vi "dsdll_output_set_volume.vi"(8 "error in":errorcluster, 9 "panning (0: balanced)":i32 min=-10000 max=10000 step=1, 10 "volume (0: full)":i32 min=-10000 max=0 step=1, 11 "dsdll instance in":T1={"dsdll path"=path "E:/LVprog/DirectSoundDLL/dsdll.dll", "dsdll handle"=[], "output devices"=[], "capture devices"=[]}) -> (0 "error out":errorcluster, 3 "dsdll instance out":T1)   [LabVIEW 2020, in "dsdll.lvlib"]
doc: "Call to set volume and panning of the playback. 'volume' range is {-10000 to 0}, where -10000 is equal to -100dB and 0 is 0dB (max volume). 'panning' range is {-10000 to +10000} where 10000 is equal to 100dB."
uses:
  dsdll.lvlib
  dsdll_instance.ctl
  dsdll_device_record.ctl
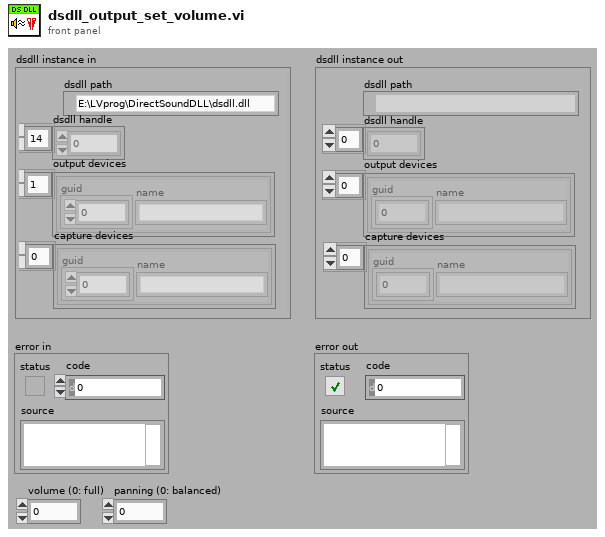
[diagram p1: front panel]
types:
  T1 = typedef "dsdll.lvlib/dsdll_instance.ctl" = cluster{"dsdll path":path, "dsdll handle":u8[], "output devices":T2[], "capture devices":T2[]}
  T2 = typedef "dsdll.lvlib/dsdll_device_record.ctl" = cluster{"guid":u8[], "name":string}
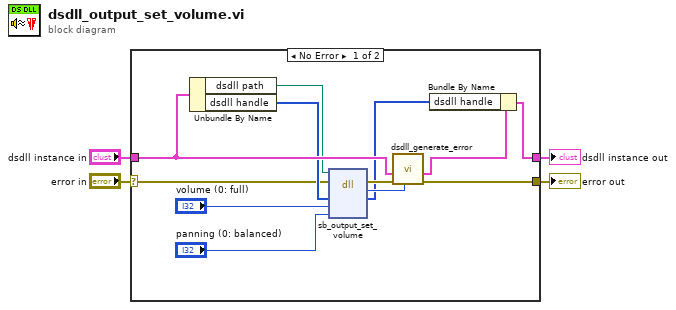
[diagram p0: block diagram]
diagram:
  n1 = case shown="No Error" "error in" {
    selector: "error in" -> [w7 w17]
    tunnel: "dsdll instance in" -> [w14 w18]
    tunnel: [w11 w17] -> w3
    tunnel: [w8 w18] -> w4
    frame No Error {
      n2 = Unbundle By Name(w14) -> ("dsdll path"=w13:path, "dsdll handle"=w12:u8[])
      n3 = dll-call lib="dsdll.dll" fn="sb_output_set_volume" ("sb_get_handle_size()")(path in=w13, error in=w7, "handle"=w12, "volume"="volume (0: full)", "panning"="panning (0: balanced)") -> (error out=w16:errorcluster, "error"=w15:i32, "handle"=w9:u8[])  [unwired: 3 in, 1 out]
      n4 = call "dsdll_generate_error.vi"("error code"=w15, "error in"=w16, "dsdll instance in"=w14) -> ("error out"=w11:errorcluster, "dsdll instance out"=w10:T1)  [unwired: 6 in, 1 out]
      n5 = Bundle By Name(cluster=w10, "dsdll handle"=w9) -> (w8:T1)
    }
    frame Error {
    }
  }
  "error out" <- w3
  "dsdll instance out" <- w4
